vi "Exercice exemple guidé 1.vi"() -> ()   [LabVIEW 2018]
panel:
  out "c":dbl
  in  "b":dbl
  in  "a":dbl
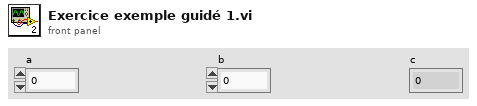
[diagram p1: front panel]
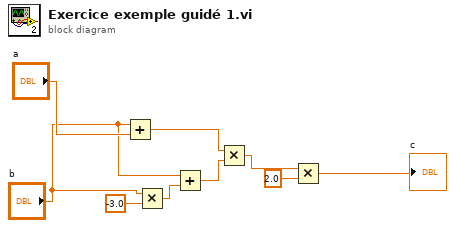
[diagram p0: block diagram]
diagram:
  n1 = Add(x="b", y="a") -> (x+y=w8:dbl)
  n2 = Multiply(x="b", y=-3.0) -> (x*y=w3:dbl)
  n3 = Add(x="b", y=w3) -> (x+y=w1:dbl)
  n4 = Multiply(x=w8, y=w1) -> (x*y=w7:dbl)
  n5 = Multiply(x=w7, y=2.0) -> (x*y=→"c":dbl)
